vi "Get Queue Ref.vi"(8 "error in (no error)":errorcluster) -> (0 "error out":errorcluster, 3 "Queue Ref":refnum<queue>)   [LabVIEW 2022 SP3]
doc: "Issues a command to the Process module by enqueuing into the Process module queue."
uses:
  Message.ctl
  Command.ctl
panel:
  # "Development\ncontrols/indicators useful for development and testing, but which are not outputs of the VI"
  # "Input\nInputs to the VI"
  # "Output\nOutputs of the VI"
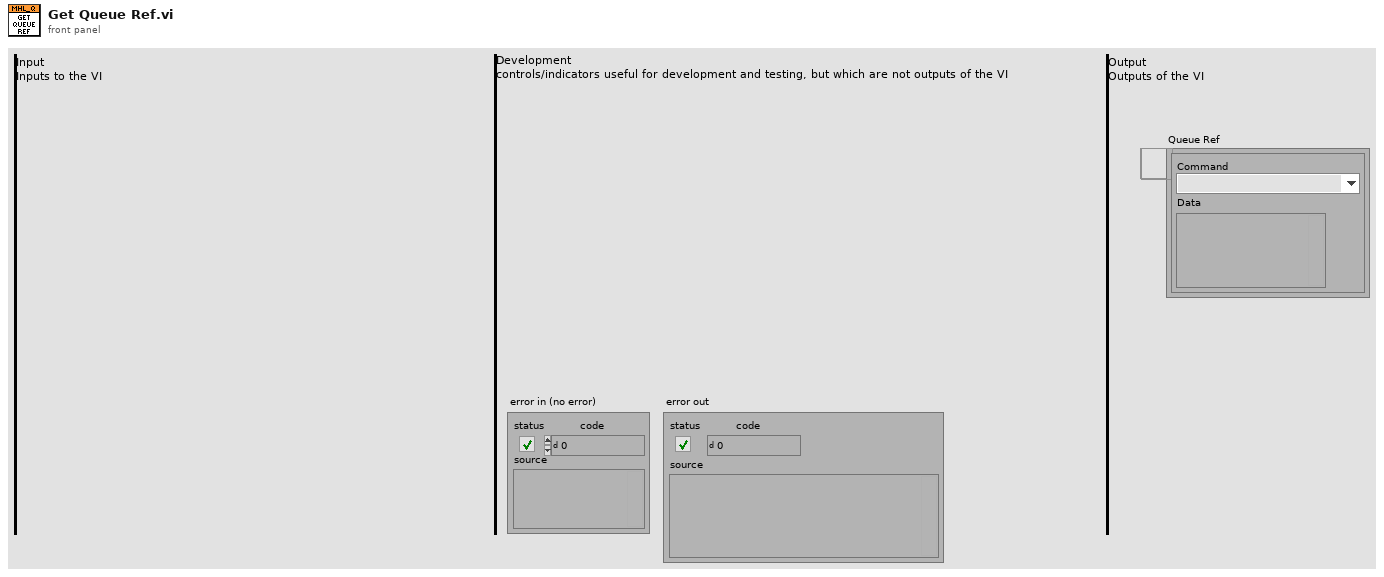
[diagram p1: front panel]
types:
  T1 = typedef "Message.ctl" = cluster{"Command":T2, "Data":variant}
  T2 = typedef "Command.ctl" = enum16{"Init Module", "Close Module", "Local Error Handler", "Command 1 (replace me)", "Command 2 (replace me)", "Command 3 (replace me)"}
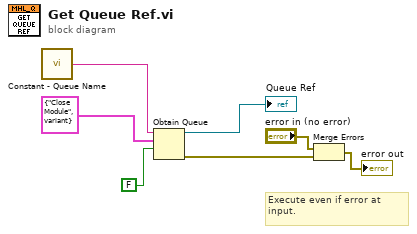
[diagram p0: block diagram]
diagram:
  # "Execute even if error at input."
  n1 = call "Constant - Queue Name.vi"() -> ("Queue Name"=w5:string)
  n2 = Obtain Queue(name (unnamed)=w5, element data type=T1 {"Command"=enum."Close Module", "Data"=variant} ("Queue Message"), create if not found? (T)=FALSE) -> (queue out=→"Queue Ref":refnum<queue>, error out=w7:errorcluster)  [unwired: 2 in, 1 out]
  n3 = Merge Errors("error in (no error)", w7) -> (→"error out":errorcluster)
